vi "RSNRPZ Set Dropout Time.vi"(8 "error in (no error)":errorcluster, 9 "Dropout Time (0.0 s)":dbl format="%^.3e", 10 "Channel (1)":i32=1, 11 "VISA session":refnum<visa-resource-name> caption="VISA resource name") -> (0 "error out":errorcluster, 3 "dup VISA session":refnum<visa-resource-name> caption="VISA resource name")   [LabVIEW 2010]
doc: "This VI defines the dropout time value. With a positive (negative) trigger slope, the dropout time is the minimum time for which the signal must be below (above) the power level defined by rsnrpz_trigger_setLevel and rsnrpz_trigger_setHysteresis before triggering can occur again. As with the Holdoff parameter, unwanted trigger events can be excluded. The set dropout time only affects the internal trigger source.\nThe dropout time parameter is useful when dealing with, for example, GSM signals with several active slots.\n\nRemote-control command(s):\nTRIGger:DTIMe"
uses:
  rsnrpz_32.dll
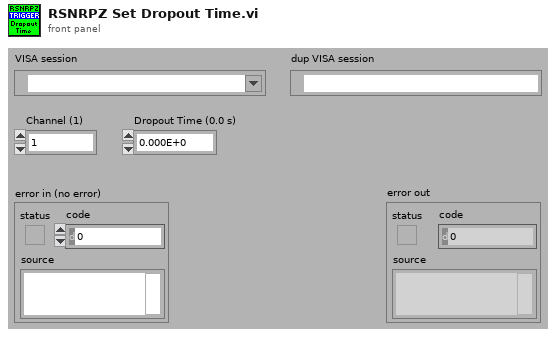
[diagram p1: front panel]
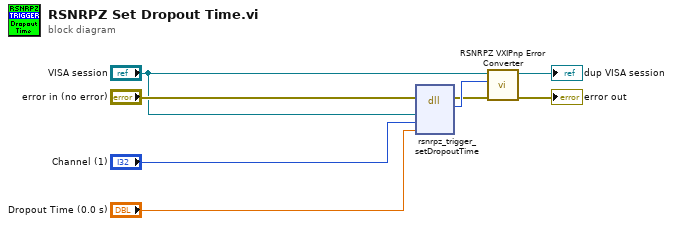
[diagram p0: block diagram]
diagram:
  n1 = dll-call lib="rsnrpz_32.dll" fn="rsnrpz_trigger_setDropoutTime"(error in="error in (no error)", "Instrument Handle"="VISA session", "Channel"="Channel (1)", "Dropout Time"="Dropout Time (0.0 s)") -> (error out=w5:errorcluster, "Status"=w8:i32)  [unwired: 5 in, 1 out]
  n2 = call <instrlib>:"RSNRPZ VXIPnp Error Converter.vi"("error in"=w5, "VXIPnp error code"=w8, "VISA session"="VISA session") -> ("error out"=→"error out":errorcluster, "dup VISA session"=→"dup VISA session":refnum<visa-resource-name>)  [unwired: 7 in]
